vi "secuencia.vi"   [LabVIEW 2020]
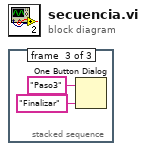
[diagram p0: block diagram]
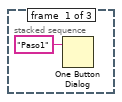
[diagram p2: hidden frame]
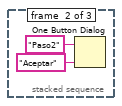
[diagram p3: hidden frame]
diagram:
  n1 = stacked-sequence {
    frame #0 {
      n2 = One Button Dialog(message="Paso1") -> ()  [unwired: 1 in, 1 out]
    }
    frame #1 {
      n3 = One Button Dialog(message="Paso2", button name ("OK")="Aceptar") -> ()  [unwired: 1 out]
    }
    frame #2 {
      n4 = One Button Dialog(message="Paso3", button name ("OK")="Finalizar") -> ()  [unwired: 1 out]
    }
  }
